vi "Enable myRIO Support.vi"(8 "Error In":errorcluster, 11 "myRIO Support":enum16{"Enabled", "Disabled"}(ring)) -> (0 "Error Out":errorcluster)   [LabVIEW 2011, in "LVH-LINX.lvlib"]
uses:
  <vilib>/LabVIEW Hacker/LINX/LVH-LINX.lvlib
  <vilib>/Utility/traverseref.llb/TRef TravTarget.ctl
  <vilib>/Utility/traverseref.llb/VI Scripting - Traverse.lvlib
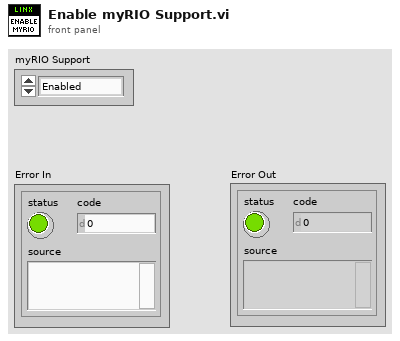
[diagram p1: front panel]
types:
  T1 = typedef "TRef TravTarget.ctl" = enum16{"FP", "BD", "Other"}
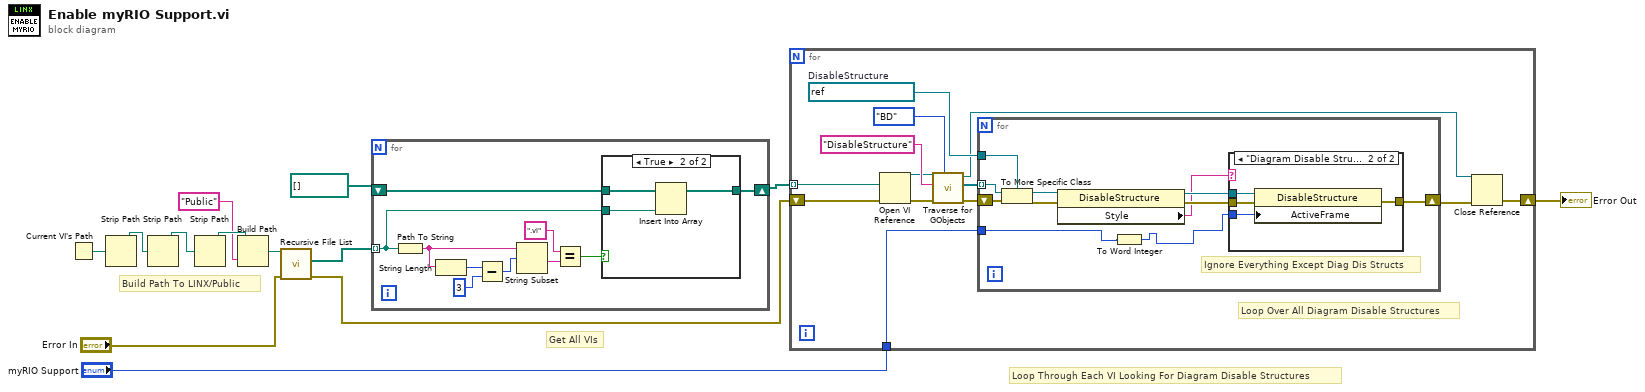
[diagram p0: block diagram]
diagram:
  # "Loop Through Each VI Looking For Diagram Disable Structures"
  # "Get All VIs"
  # "Build Path To LINX/Public"
  n1 = Current VI's Path() -> (path=w13:path)
  n2 = Strip Path(path=w13) -> (stripped path=w10:path)  [unwired: 1 out]
  n3 = Strip Path(path=w10) -> (stripped path=w9:path)  [unwired: 1 out]
  n4 = Strip Path(path=w9) -> (stripped path=w12:path)  [unwired: 1 out]
  n5 = Build Path(base path=w12, name or relative path="Public") -> (appended path=w2:path)
  n6 = call <vilib>:"Recursive File List.vi"("error in (no error)"="Error In", "Folder Path"=w2) -> ("error out"=w5:errorcluster, "All Files in Dir"=w7:path[])  [unwired: 5 in, 3 out]
  n7 = for {
    tunnel: w7 -> [w21] mode=indexing
    shift-right: [w22] -> w6
    shift-left: path[] [] ("array") -> [w23]
    n8 = Path To String(path=w21) -> (string=w20:string)
    n9 = String Length(string=w20) -> (length=w19:i32)
    n10 = Subtract(x=w19, y=3) -> (x-y=w17:i32)
    n11 = String Subset(string=w20, offset (0)=w17) -> (substring=w16:string)  [unwired: 1 in]
    n12 = Equal?(x=".vi", y=w16) -> (x = y?=w14:bool)
    n13 = case shown="True" w14 {
      tunnel: w21 -> [_ w27]
      tunnel: w23 -> [w24 w26]
      tunnel: [w24 w25] -> w22
      frame False {
      }
      frame True {
        n14 = Insert Into Array(array=w26, new element=w27) -> (w25:path[])  [unwired: 1 in]
      }
    }
  }
  n15 = for {
    tunnel: w6 -> [w34] mode=indexing
    shift-right: [w29] -> w4
    shift-left: w5 -> [w33]
    tunnel: "myRIO Support" -> [w31]
    w38 = refnum<vi> refnum  # DisableStructure
    # "Loop Over All Diagram Disable Structures"
    n16 = Open VI Reference(vi path=w34, error in (no error)=w33) -> (vi reference=w35:refnum<vi>, error out=w40:errorcluster)  [unwired: 4 in]
    n17 = call <vilib>:"Traverse for GObjects.vi"("Traverse Target"=TRef_TravTarget."BD", "error in (no error)"=w40, "Class Name"="DisableStructure", "VI Refnum"=w35) -> ("error out"=w39:errorcluster, "References"=w32:refnum<vi>[], "dup VI Refnum"=w28:refnum<vi>)  [unwired: 4 in, 1 out]
    n18 = for {
      tunnel: w38 -> [w50]
      tunnel: w32 -> [w49] mode=indexing
      shift-right: [w48] -> w30
      shift-left: w39 -> [w51]
      tunnel: w31 -> [w42]
      # "Ignore Everything Except Diag Dis Structs"
      n19 = To More Specific Class(target class=w50, reference=w49, error in=w51) -> (specific class reference=w45:refnum<vi>, error out=w47:errorcluster)
      n20 = property class="DisableStructure"(reference=w45, error in=w47) -> (reference out=w44:refnum<vi>, error out=w46:errorcluster, "Style"=w43:string)
      n21 = To Word Integer(number=w42) -> (16bit integer=w41:i16)
      n22 = case shown="\"Diagram Disable Structure\"" w43 {
        tunnel: w41 -> [_ w56]
        tunnel: [w52 w55] -> w48
        tunnel: w46 -> [w52 w54]
        tunnel: w44 -> [_ w53]
        frame Default {
        }
        frame "Diagram Disable Structure" {
          n23 = property class="DisableStructure"(reference=w53, error in=w54, "ActiveFrame"=w56) -> (error out=w55:errorcluster)  [unwired: 1 out]
        }
      }
    }
    n24 = Close Reference(reference=w28, error in (no error)=w30) -> (error out=w29:errorcluster)
  }
  "Error Out" <- w4
